vi "GH-311.vi"(8 "Error In":errorcluster, 10 "SIG Pin (DIO)":u8, 11 "LINX Resource":T1) -> (0 "Error Out":errorcluster, 1 "Inches":dbl, 2 "Centimeters":dbl, 3 "LINX Resource":T1)   [LabVIEW 2013, in "LVH-LINX.lvlib" / "Ultrasonic.lvlib"]
doc: "Read distance using the GH-311 ultrasonic distance sensor."
uses:
  <vilib>/LabVIEW Hacker/LINX/Public/Sensors/Ultrasonic/Ultrasonic.lvlib
  <vilib>/LabVIEW Hacker/LINX/Private/Type Defs/LINX Ref.ctl
  <vilib>/LabVIEW Hacker/LINX/Private/Type Defs/Platform.ctl
  <vilib>/LabVIEW Hacker/LINX/Private/Type Defs/Interface.ctl
  <vilib>/LabVIEW Hacker/LINX/Private/Device/Type Defs/LINX Device Config.ctl
  <vilib>/LabVIEW Hacker/LINX/Private/Device/Type Defs/TCP Config.ctl
  <vilib>/LabVIEW Hacker/LINX/Private/Type Defs/Device Family.ctl
  <vilib>/LabVIEW Hacker/LINX/LVH-LINX.lvlib
  <vilib>/LabVIEW Hacker/LINX/Private/Device/Device.lvlib
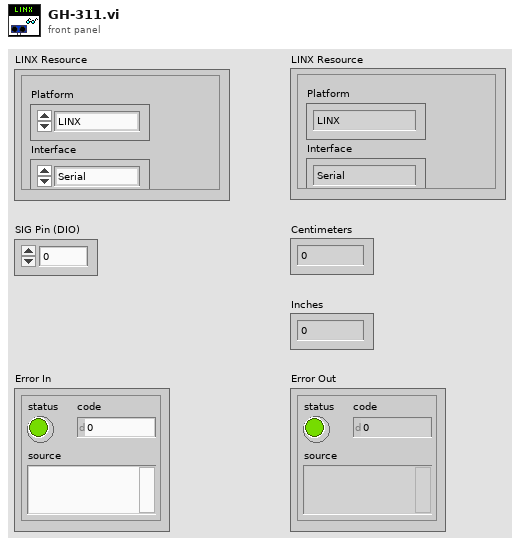
[diagram p1: front panel]
types:
  T1 = typedef "LVH-LINX.lvlib/LINX Ref.ctl" = cluster{"Platform":T2, "Interface":T3, "LINX Device Config":T4}
  T2 = typedef "LVH-LINX.lvlib/Platform.ctl" = enum16{"LINX", "myRIO"}
  T3 = typedef "LVH-LINX.lvlib/Interface.ctl" = enum16{"Serial", "TCP"}
  T4 = typedef "LVH-LINX.lvlib/Device.lvlib/LINX Device Config.ctl" = cluster{"Interface":T3, "COM Port":refnum<visa-resource-name>, "TCP Configuration":T5, "Device Family":T6, "Device ID":u8, "Device Name":string, "TCP Ref":refnum<k5>}
  T5 = typedef "LVH-LINX.lvlib/Device.lvlib/TCP Config.ctl" = cluster{"IP Address":string, "Port":u16}
  T6 = typedef "LVH-LINX.lvlib/Device Family.ctl" = enum8{"National Instruments", "Digilent", "Arduino"}
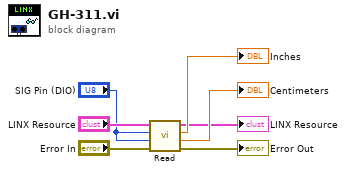
[diagram p0: block diagram]
diagram:
  n1 = call <vilib>:"Read.vi"("Error In"="Error In", "DO Channel"="SIG Pin (DIO)", "DI Channel"="SIG Pin (DIO)", "LINX Resource"="LINX Resource") -> ("Error Out"=→"Error Out":errorcluster, "Centimeters"=→"Centimeters":dbl, "Inches"=→"Inches":dbl, "LINX Resource"=→"LINX Resource":T1)  [unwired: 4 in]
